vi "CheckPressureStability.vi"(8 "error in":errorcluster, 11 "S1 in":refnum<class "S3.lvclass">) -> (0 "error out":errorcluster, 3 "S1 out":refnum<class "S3.lvclass">)   [LabVIEW 2018, in "S3.lvclass"]
uses:
  S3.lvclass
  S3.lvclass/S3.ctl
  Public Controls/Outputs.ctl
  Public Controls/ReportHeader.ctl
  IO/IO.lvclass
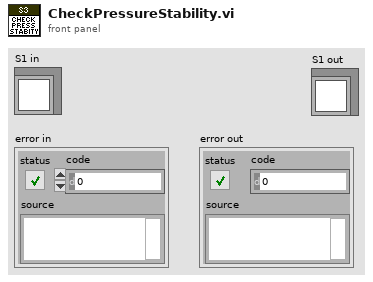
[diagram p1: front panel]
types:
  T1 = typedef "S3.lvclass/Outputs.ctl" = cluster{"LO P":bool, "HI P":bool, "Z3Vent":bool, "V2 Vent":bool, "IsLidLocked":bool}
  T2 = typedef "S3.lvclass/ReportHeader.ctl" = string
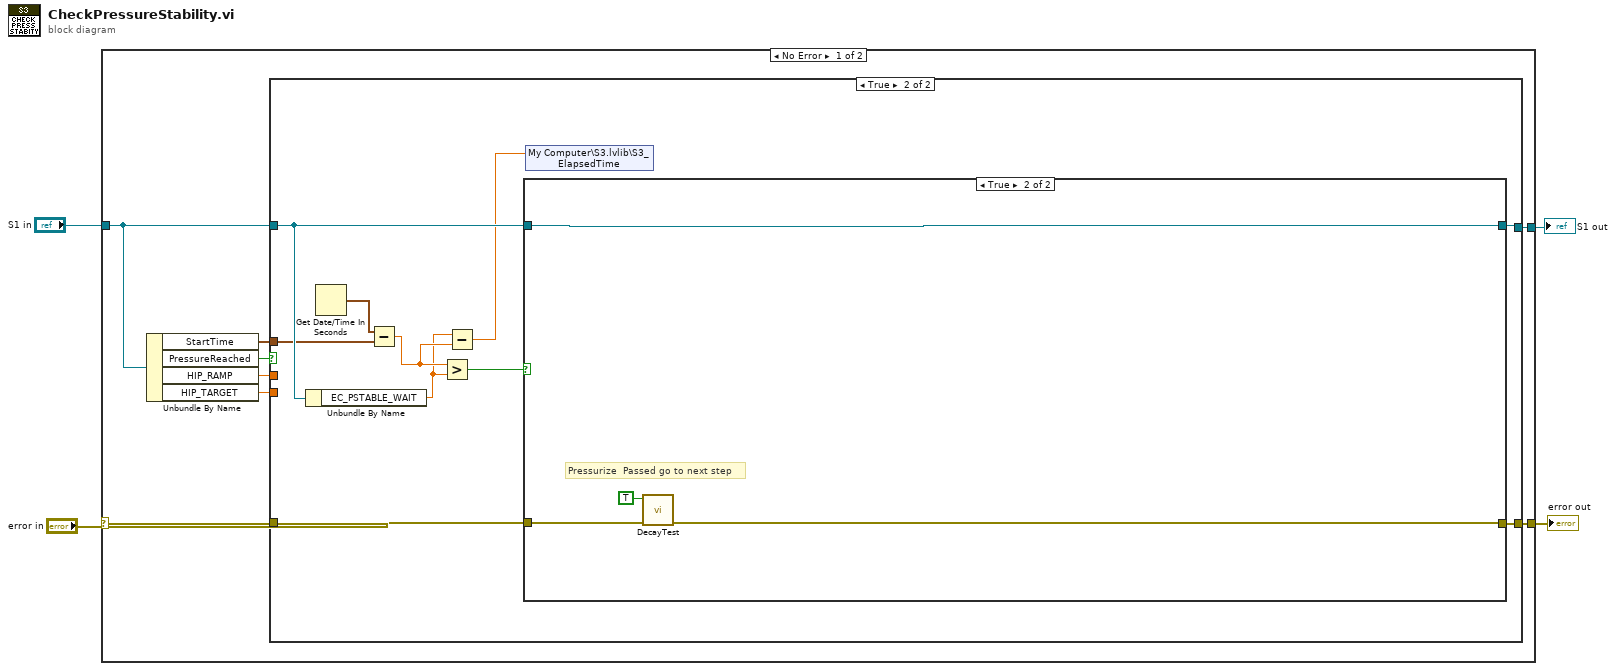
[diagram p0: block diagram]
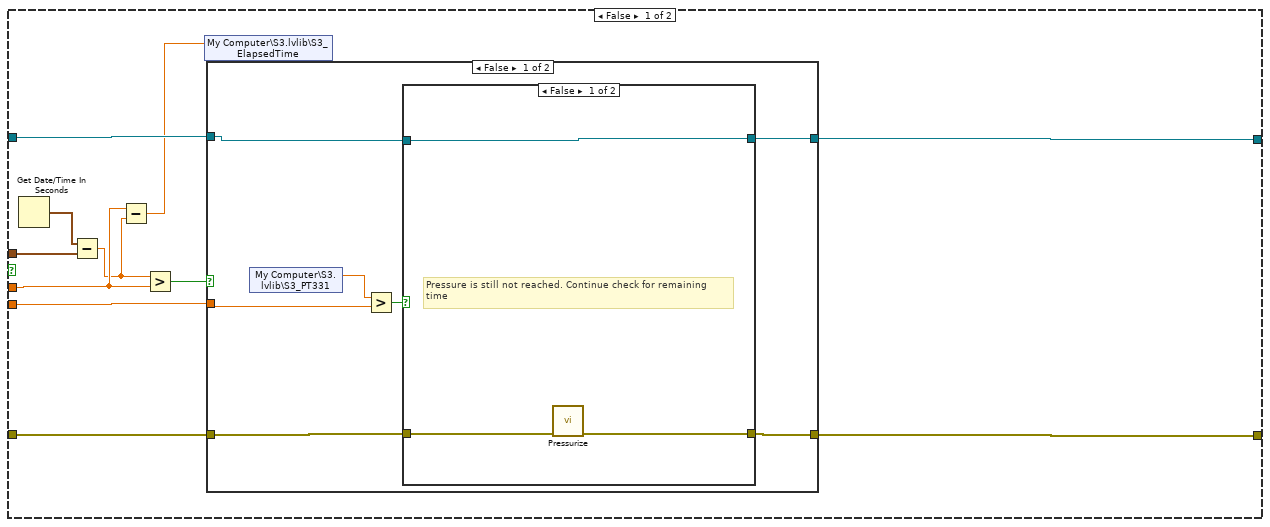
[diagram p2: hidden frame]
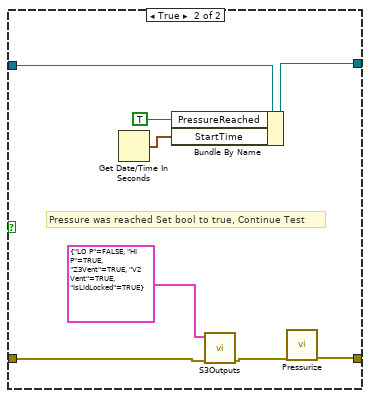
[diagram p3: hidden frame]
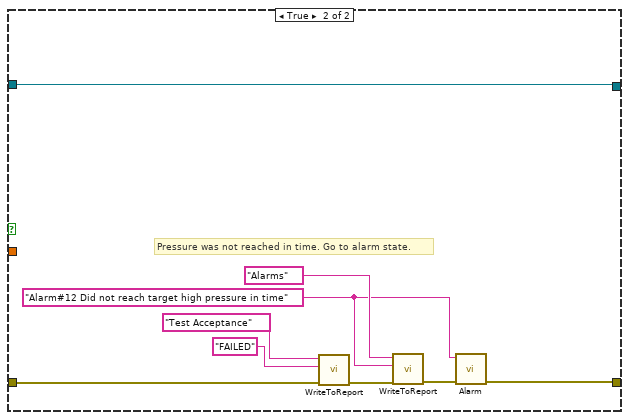
[diagram p4: hidden frame]
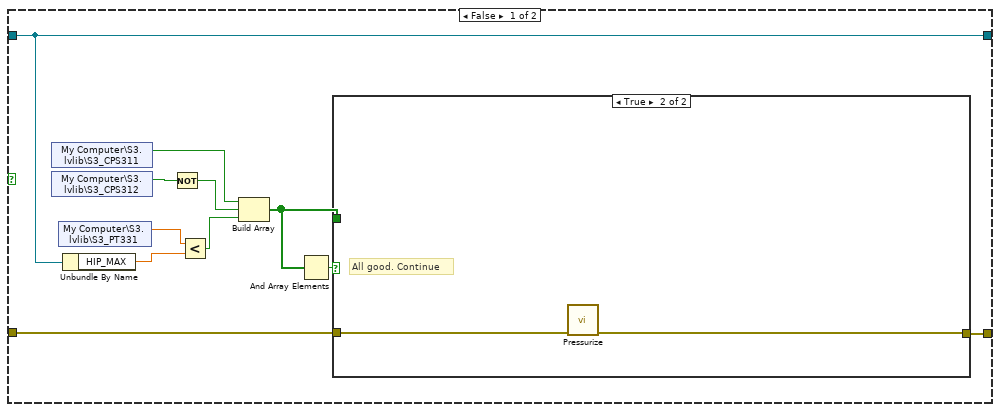
[diagram p5: hidden frame]
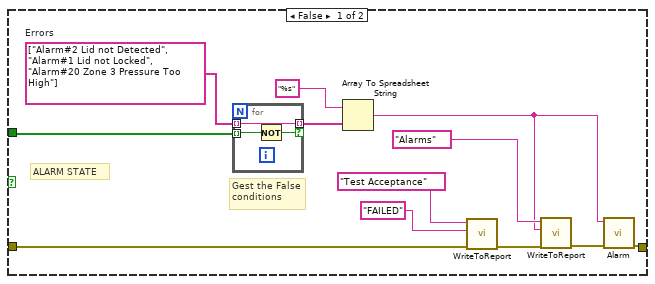
[diagram p6: hidden frame]
diagram:
  n1 = case shown="No Error" "error in" {
    selector: "error in" -> [w12 w94]
    tunnel: [w9 w94] -> w4
    tunnel: "S1 in" -> [w8 w93]
    tunnel: [w10 w93] -> w1
    frame No Error {
      n2 = Unbundle By Name(w8) -> ("StartTime"=w7:timestamp, "PressureReached"=w11:bool, "HIP_RAMP"=w6:dbl, "HIP_TARGET"=w5:dbl)
      n3 = case shown="True" w11 {
        tunnel: w12 -> [w21 w60]
        tunnel: [w19 w59] -> w9
        tunnel: w7 -> [w22 w54]
        tunnel: w8 -> [w18 w58]
        tunnel: [w17 w57] -> w10
        tunnel: w6 -> [w16 _]
        tunnel: w5 -> [w13 _]
        frame False {
          n4 = Get Date/Time In Seconds() -> (seconds since 1Jan1904=w23:timestamp)
          n5 = Subtract(x=w23, y=w22) -> (x-y=w15:dbl)
          n6 = Subtract(x=w16, y=w15) -> (x-y=w14:dbl)
          n7 = Greater?(x=w15, y=w16) -> (0:w20:bool)
          n8 = shared-variable "My Computer\\S3.lvlib\\S3_ElapsedTime"(w14) -> ()  [unwired: 1 in, 1 out]
          n9 = case shown="False" w20 {
            tunnel: w21 -> [w26 w45]
            tunnel: [w25 w47] -> w19
            tunnel: w18 -> [w28 w44]
            tunnel: [w27 w44] -> w17
            tunnel: w13 -> [w24 _]
            frame False {
              n10 = shared-variable "My Computer\\S3.lvlib\\S3_PT331"() -> (w30:dbl)  [unwired: 1 in, 1 out]
              n11 = Greater?(x=w30, y=w24) -> (0:w29:bool)
              n12 = case shown="False" w29 {
                tunnel: w28 -> [w33 w41]
                tunnel: [w33 w40] -> w27
                tunnel: w26 -> [w32 w35]
                tunnel: [w31 w38] -> w25
                frame False {
                  # "Pressure is still not reached. Continue check for remaining\ntime"
                  n13 = call "Pressurize.vi"("error in"=w32) -> ("error out"=w31:errorcluster)  [unwired: 10 in]
                }
                frame True {
                  # "Pressure was reached Set bool to true, Continue Test"
                  n14 = Get Date/Time In Seconds() -> (seconds since 1Jan1904=w37:timestamp)
                  n15 = Bundle By Name(cluster=w41, "PressureReached"=TRUE ("PT111ReachedPressure"), "StartTime"=w37) -> (w40:refnum<class "S3.lvclass">)
                  n16 = call "S3Outputs.vi"("error in"=w35, "SIOutputs"=T1 {"LO P"=FALSE, "HI P"=TRUE, "Z3Vent"=TRUE, "V2 Vent"=TRUE, "IsLidLocked"=TRUE}) -> ("error out"=w34:errorcluster)  [unwired: 9 in]
                  n17 = call "Pressurize.vi"("error in"=w34) -> ("error out"=w38:errorcluster)  [unwired: 10 in]
                }
              }
            }
            frame True {
              w43 = "Alarm#12 Did not reach target high pressure in time" ("Value")
              # "Pressure was not reached in time. Go to alarm state."
              n18 = call "WriteToReport.vi"("error in"=w45, "Value"="FAILED", "Header"=T2 "Test Acceptance") -> ("error out"=w50:errorcluster)  [unwired: 8 in]
              n19 = call "WriteToReport.vi"("error in"=w50, "Value"=w43, "Header"="Alarms") -> ("error out"=w48:errorcluster)  [unwired: 8 in]
              n20 = call "Alarm.vi"("error in"=w48, "Alarm"=w43) -> ("error out"=w47:errorcluster)  [unwired: 9 in]
            }
          }
        }
        frame True {
          n21 = Unbundle By Name(w58) -> ("EC_PSTABLE_WAIT"=w53:dbl)
          n22 = Get Date/Time In Seconds() -> (seconds since 1Jan1904=w56:timestamp)
          n23 = Subtract(x=w56, y=w54) -> (x-y=w55:dbl)
          n24 = Greater?(x=w55, y=w53) -> (0:w52:bool)
          n25 = Subtract(x=w53, y=w55) -> (x-y=w51:dbl)
          n26 = case shown="True" w52 {
            tunnel: [w71 w92] -> w59
            tunnel: w60 -> [w65 w91]
            tunnel: w58 -> [w62 w90]
            tunnel: [w62 w90] -> w57
            frame False {
              n27 = shared-variable "My Computer\\S3.lvlib\\S3_CPS311"() -> (w67:bool)  [unwired: 1 in, 1 out]
              n28 = shared-variable "My Computer\\S3.lvlib\\S3_CPS312"() -> (w66:bool)  [unwired: 1 in, 1 out]
              n29 = shared-variable "My Computer\\S3.lvlib\\S3_PT331"() -> (w63:dbl)  [unwired: 1 in, 1 out]
              n30 = Unbundle By Name(w62) -> ("HIP_MAX"=w61:dbl)
              n31 = Not(x=w66) -> (.not. x?=w64:bool)
              n32 = Less?(x=w63, y=w61) -> (x < y?=w70:bool)
              n33 = Build Array(w67, w64, w70) -> (w68:bool[])
              n34 = And Array Elements(Boolean array=w68) -> (logical AND=w69:bool)
              n35 = case shown="True" w69 {
                tunnel: w65 -> [w78 w88]
                tunnel: [w80 w87] -> w71
                tunnel: w68 -> [w77 _]
                frame False {
                  w76 = string[] ["Alarm#2 Lid not Detected", "Alarm#1 Lid not Locked", "Alarm#20 Zone 3 Pressure Too High"]  # Errors
                  # "ALARM STATE"
                  # "Gest the False\nconditions"
                  n36 = for {
                    tunnel: w77 -> [w85] mode=indexing
                    tunnel: w76 -> [w86] mode=indexing
                    tunnel: [w86] -> w75 mode=indexing if=w84
                    n37 = Not(x=w85) -> (.not. x?=w84:bool)
                  }
                  n38 = Array To Spreadsheet String(array=w75, 3:"%s" ("format string")) -> (spreadsheet string=w73:string)  [unwired: 1 in]
                  n39 = call "WriteToReport.vi"("error in"=w78, "Value"="FAILED", "Header"=T2 "Test Acceptance") -> ("error out"=w83:errorcluster)  [unwired: 8 in]
                  n40 = call "WriteToReport.vi"("error in"=w83, "Value"=w73, "Header"="Alarms") -> ("error out"=w81:errorcluster)  [unwired: 8 in]
                  n41 = call "Alarm.vi"("error in"=w81, "Alarm"=w73) -> ("error out"=w80:errorcluster)  [unwired: 9 in]
                }
                frame True {
                  # "All good. Continue"
                  n42 = call "Pressurize.vi"("error in"=w88) -> ("error out"=w87:errorcluster)  [unwired: 10 in]
                }
              }
            }
            frame True {
              # "Pressurize  Passed go to next step"
              n43 = call "DecayTest.vi"("error in"=w91, "FirstCall(F)"=TRUE) -> ("error out"=w92:errorcluster)  [unwired: 9 in]
            }
          }
          n44 = shared-variable "My Computer\\S3.lvlib\\S3_ElapsedTime"(w51) -> ()  [unwired: 1 in, 1 out]
        }
      }
    }
    frame Error {
    }
  }
  "error out" <- w4
  "S1 out" <- w1
